vi "Meas Init UI.vi"(8 "error in (no error)":errorcluster, 11 "UI Data in":T1) -> (0 "error out":errorcluster)   [LabVIEW 2014]
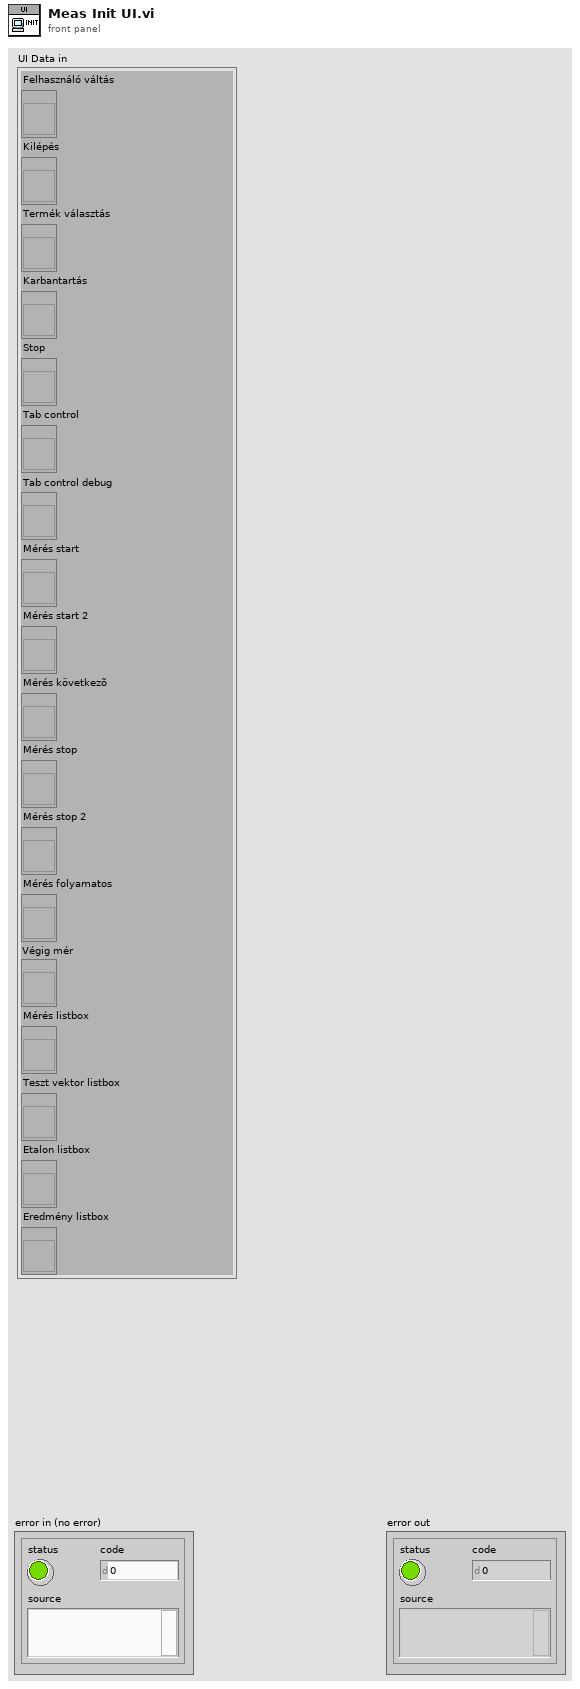
[diagram p1: front panel]
types:
  T1 = typedef "Fõképernyõ references.ctl" = cluster{"Felhasználó váltás":refnum<vi>, "Kilépés":refnum<vi>, "Termék választás":refnum<vi>, "Karbantartás":refnum<vi>, "Stop":refnum<vi>, "Tab control":refnum<vi>, "Tab control debug":refnum<vi>, "Mérés start":refnum<vi>, "Mérés start 2":refnum<vi>, "Mérés következõ":refnum<vi>, "Mérés stop":refnum<vi>, "Mérés stop 2":refnum<vi>, "Mérés folyamatos":refnum<vi>, "Végig mér":refnum<vi>, "Mérés listbox":refnum<vi>, "Teszt vektor listbox":refnum<vi>, "Etalon listbox":refnum<vi>, "Eredmény listbox":refnum<vi>}
  T2 = enum8{"Enabled", "Disabled", "Disabled and Grayed Out"}
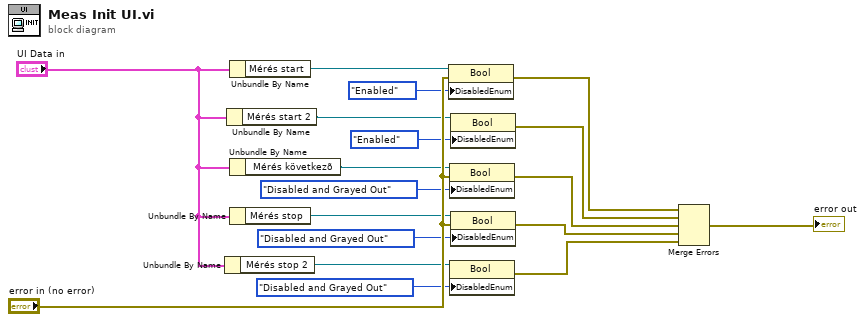
[diagram p0: block diagram]
diagram:
  n1 = Unbundle By Name("UI Data in") -> ("Mérés stop 2"=w4:refnum<vi>)
  n2 = Unbundle By Name("UI Data in") -> ("Mérés start 2"=w9:refnum<vi>)
  n3 = Unbundle By Name("UI Data in") -> ("Mérés start"=w12:refnum<vi>)
  n4 = Unbundle By Name("UI Data in") -> ("Mérés következõ"=w14:refnum<vi>)
  n5 = Unbundle By Name("UI Data in") -> ("Mérés stop"=w15:refnum<vi>)
  n6 = property on="Property Node" class="Bool"(reference=w12, error in="error in (no error)", "DisabledEnum"=T2."Enabled" ("Disabled")) -> (error out=w8:errorcluster)  [unwired: 1 out]
  n7 = property on="Property Node" class="Bool"(reference=w14, error in="error in (no error)", "DisabledEnum"=T2."Disabled and Grayed Out" ("Disabled")) -> (error out=w6:errorcluster)  [unwired: 1 out]
  n8 = property on="Property Node" class="Bool"(reference=w4, "DisabledEnum"=T2."Disabled and Grayed Out" ("Disabled")) -> (error out=w1:errorcluster)  [unwired: 1 in, 1 out]
  n9 = property on="Property Node" class="Bool"(reference=w9, "DisabledEnum"=T2."Enabled" ("Disabled")) -> (error out=w7:errorcluster)  [unwired: 1 in, 1 out]
  n10 = property on="Property Node" class="Bool"(reference=w15, error in="error in (no error)", "DisabledEnum"=T2."Disabled and Grayed Out" ("Disabled")) -> (error out=w5:errorcluster)  [unwired: 1 out]
  n11 = Merge Errors(w8, w7, w6, w5, w1) -> (→"error out":errorcluster)
